vi "movement forward by santimeters.vi"() -> ()   [LabVIEW 2017]
uses:
  <vilib>/myRIO/Common/Instrument Driver Framework/Utilities/typedefs/FPGA Ref Manager Action Enum.ctl
  <vilib>/myRIO/Common/Instrument Driver Framework/myRIO v1.0/Encoder/typedefs/Encoder Signal Mode.ctl
  <vilib>/myRIO/Instrument Drivers/Onboard IO/Encoder/typedefs/Encoder Reference.ctl
  <vilib>/myRIO/Common/Instrument Driver Framework/Utilities/typedefs/myRIO Generic Hardware Reference.ctl
  <vilib>/myRIO/Common/Instrument Driver Framework/Utilities/typedefs/Hardware Version Enum.ctl
  <vilib>/myRIO/Common/Instrument Driver Framework/Utilities/typedefs/myRIO v1.0 Reference.ctl
  <vilib>/myRIO/Common/Instrument Driver Framework/Utilities/typedefs/Generic FPGA Reference.ctl
  <vilib>/myRIO/Common/Instrument Driver Framework/myRIO v1.0/Encoder/typedefs/Encoder Channels Enum.ctl
  <vilib>/myRIO/Common/Instrument Driver Framework/myRIO v1.0/Encoder/typedefs/Encoder Configuration v1.0.ctl
  <vilib>/userdefined/High Color/nirio_resource_hc.ctl
  <vilib>/myRIO/Instrument Drivers/Onboard IO/I2C/typedefs/I2C Reference.ctl
  <vilib>/myRIO/Common/Instrument Driver Framework/myRIO v1.0/I2C/typedefs/I2C Channels Enum.ctl
  <vilib>/myRIO/Instrument Drivers/Onboard IO/I2C/typedefs/I2C Configuration.ctl
  <vilib>/myRIO/Instrument Drivers/Onboard IO/I2C/typedefs/I2C Transfer Rate.ctl
  <vilib>/myRIO/Common/Instrument Driver Framework/Utilities/vis/Is FPGA Ref Available.vi
  <vilib>/myRIO/Common/Instrument Driver Framework/myRIO v1.0/Encoder/vis/myRIO v1.1 Open Encoder.vi
  <vilib>/myRIO/Instrument Drivers/Onboard IO/Encoder/vis/Read.vi
  <vilib>/myRIO/Common/Instrument Driver Framework/myRIO v1.0/I2C/vis/myRIO v1.1 Open I2C.vi
  <vilib>/myRIO/Common/Instrument Driver Framework/Utilities/vis/Validate Channels.vi
  <vilib>/myRIO/Common/Instrument Driver Framework/myRIO v1.0/Encoder/vis/myRIO v1.0 Reserve Encoder.vi
  <vilib>/myRIO/Common/Instrument Driver Framework/myRIO v1.0/I2C/vis/myRIO v1.0 Reserve I2C.vi
  <vilib>/myRIO/Common/Instrument Driver Framework/myRIO v1.0/I2C/vis/myRIO v1.0 Close I2C.vi
  <vilib>/myRIO/Common/Instrument Driver Framework/myRIO v1.0/Encoder/vis/myRIO v1.0 Build MUX Configuration Encoder.vi
  <vilib>/myRIO/Common/Instrument Driver Framework/myRIO v1.0/Resource Manager/vis/myRIO v1.0 Reserve Channel List.vi
  <vilib>/myRIO/Common/Instrument Driver Framework/myRIO v1.0/I2C/vis/myRIO v1.0 Build MUX Configuration I2C.vi
  <vilib>/myRIO/Common/Instrument Driver Framework/myRIO v1.0/I2C/vis/myRIO v1.0 Unreserve I2C.vi
  <vilib>/myRIO/Common/Instrument Driver Framework/myRIO v1.0/Resource Manager/vis/myRIO v1.0 Create Configuration List.vi
  <vilib>/myRIO/Common/Instrument Driver Framework/myRIO v1.0/Resource Manager/vis/myRIO v1.0 Reserve Channel.vi
  <vilib>/myRIO/Common/Instrument Driver Framework/myRIO v1.0/Resource Manager/vis/myRIO v1.0 Unreserve Channel.vi
  <vilib>/myRIO/Common/Instrument Driver Framework/myRIO v1.0/Resource Manager/vis/myRIO v1.0 Unreserve Channel List.vi
  <vilib>/myRIO/Common/Instrument Driver Framework/myRIO v1.0/Resource Manager/vis/myRIO v1.0 Build Mutex Name.vi
  <vilib>/Utility/VariantDataType/GetNumericInfo.vi
  <vilib>/Utility/error.llb/Error Cluster From Error Code.vi
  <vilib>/myRIO/Common/Instrument Driver Framework/myRIO v1.0/myRIO v1.1 Open.vi
  <vilib>/myRIO/Common/Instrument Driver Framework/Utilities/vis/IO Manager.vi
  <vilib>/myRIO/Common/Instrument Driver Framework/Utilities/vis/Configuration Manager.vi
  <vilib>/myRIO/Common/Instrument Driver Framework/myRIO v1.0/Resource Manager/vis/myRIO v1.0 Configure IO.vi
  <vilib>/myRIO/Common/Instrument Driver Framework/myRIO v1.0/myRIO v1.0 Close.vi
  <vilib>/myRIO/Common/Instrument Driver Framework/myRIO v1.0/Encoder/vis/myRIO v1.0 Configure Encoder.vi
  <vilib>/myRIO/Common/Instrument Driver Framework/myRIO v1.0/Encoder/vis/myRIO v1.0 Read Encoder.vi
  <vilib>/myRIO/Common/Instrument Driver Framework/myRIO v1.0/I2C/vis/myRIO v1.0 Shutdown I2C.vi
  <vilib>/myRIO/Instrument Drivers/Onboard IO/I2C/vis/myRIO I2C Open.xnode
  <vilib>/myRIO/Express VI/Onboard IO/Encoder/Encoder Express VI.xnode
  <vilib>/myRIO/Instrument Drivers/Onboard IO/Encoder/vis/myRIO Encoder Open.xnode
  <vilib>/myRIO/Instrument Drivers/Onboard IO/I2C/I2C.lvlib
  <vilib>/myRIO/Instrument Drivers/Onboard IO/Encoder/Encoder.lvlib
panel:
  in  "range in santimeters":dbl format="%#_13g"
  out "main angle":ext
  out "error out":errorcluster
  in  "error in (no error)":errorcluster
  out "axis Z(after)":ext
  out "zero angle":ext
  out "left":dbl
  out "right":dbl
  out "axis Z(paste)":ext
  in  "Stop Button":bool
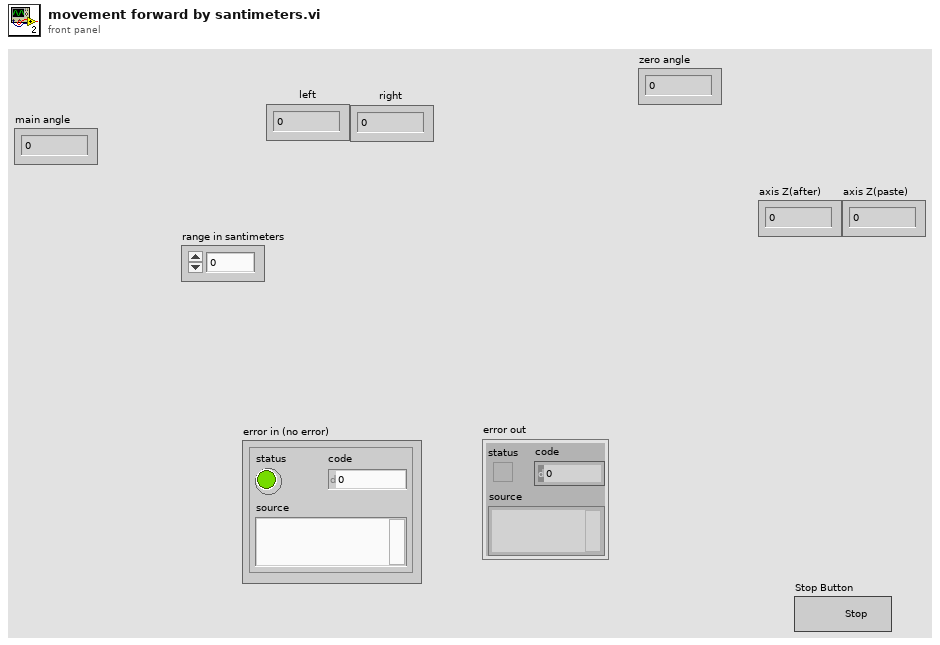
[diagram p1: front panel]
types:
  T1 = typedef "FPGA Ref Manager Action Enum.ctl" = enum16{"Get", "Set", "Reset"}
  T2 = typedef "I2C.lvlib/I2C Reference.ctl" = cluster{"myRIO Reference":T3, "I2C Channels Enum":T7, "I2C Configuration":T8}
  T3 = typedef "myRIO Generic Hardware Reference.ctl" = cluster{"myRIO Model":T4, "myRIO Hardware Reference":T5}
  T4 = typedef "Hardware Version Enum.ctl" = enum16{"Unknown", "myRIO-1900", "myRIO-1950", "roboRIO", "NI ELVIS RIO CM"}
  T5 = typedef "myRIO v1.0 Reference.ctl" = cluster{"Generic FPGA Reference":T6, "Allow multiple opens":bool}
  T6 = typedef "Generic FPGA Reference.ctl" = refnum<k20>
  T7 = typedef "I2C Channels Enum.ctl" = enum16{"Not Connected", "A/I2C", "B/I2C", "I2C/I2C"}
  T8 = typedef "I2C.lvlib/I2C Configuration.ctl" = cluster{"I2C Transfer Rate":T9}
  T9 = typedef "I2C.lvlib/I2C Transfer Rate.ctl" = enum16{"Standard mode (100 kbps)", "Fast mode (400 kbps)"}
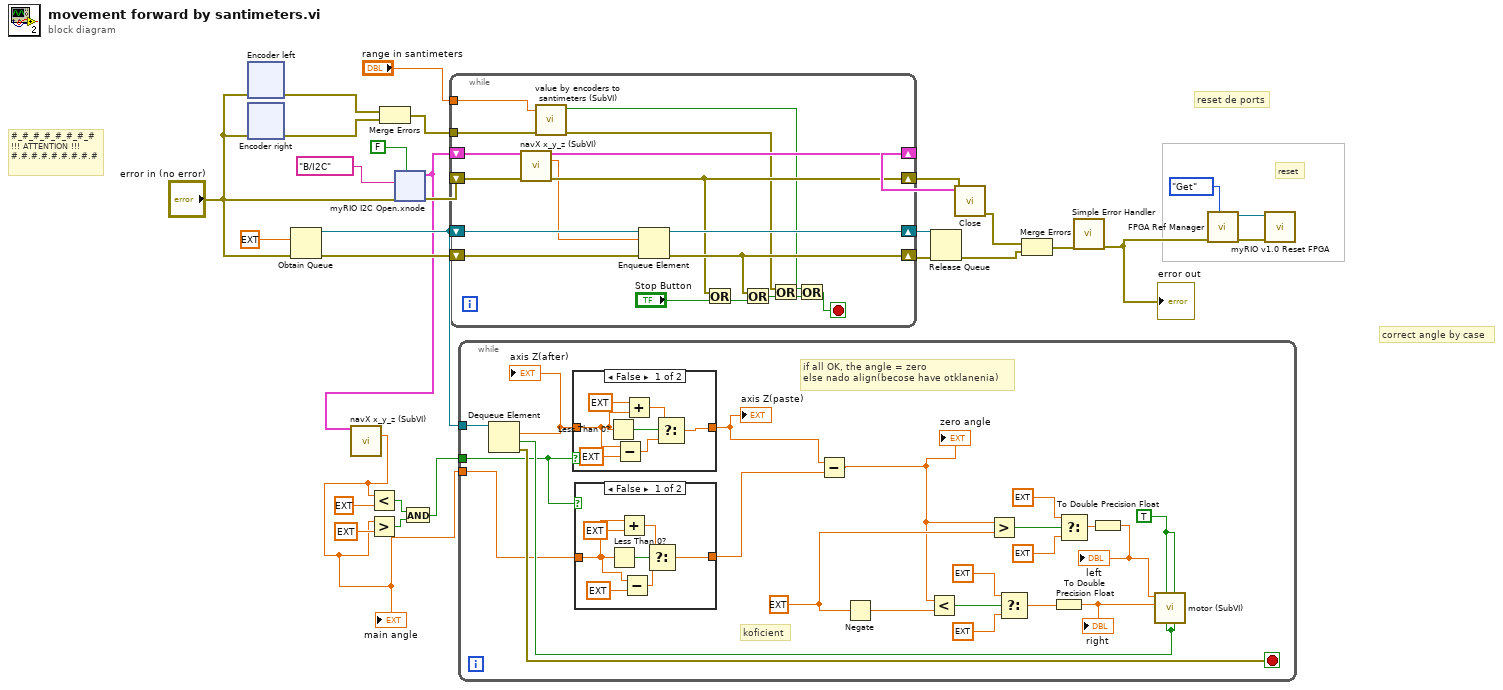
[diagram p0: block diagram]
diagram:
  # "correct angle by case"
  # "reset de ports"
  # "#_#_#_#_#_#_#_#\n!!! ATTENTION !!!\n#.#.#.#.#.#.#.#.#"
  # "reset"
  n1 = xnode ("Encoder left")("error in (no error)"="error in (no error)") -> ("error out"=w4:errorcluster)  [unwired: 1 in, 3 out]
  n2 = xnode ("Encoder right")("error in (no error)"="error in (no error)") -> ("error out"=w3:errorcluster)  [unwired: 1 in, 3 out]
  n3 = Obtain Queue(element data type=ext 0.0 ("value Z"), error in (no error)="error in (no error)") -> (queue out=w17:refnum<queue>, error out=w29:errorcluster)  [unwired: 3 in, 1 out]
  n4 = Merge Errors(w4, w3) -> (w2:errorcluster)
  n5 = xnode "myRIO I2C Open.xnode"("error in (no error)"="error in (no error)", "Allow multiple opens?"=FALSE, "Channel Name"=tag "B/I2C") -> ("error out"=w22:errorcluster, "I2C Ref Out"=w13:T2)
  n6 = call "navX x_y_z (SubVI).vi"("I2C Ref Out in"=w13) -> ("value Z"=w10:ext)  [unwired: 10 in, 4 out]
  "main angle" <- w10
  n7 = Less?(x=w10, y=ext 90.0) -> (x < y?=w8:bool)
  n8 = Greater?(x=w10, y=ext -90.0) -> (0:w11:bool)
  n9 = And(x=w8, y=w11) -> (x .and. y?=w7:bool)
  n10 = while {
    shift-right: [w41] -> w27
    shift-left: w29 -> [w46]
    shift-right: [w45] -> w28
    shift-left: w17 -> [w47]
    shift-right: [w42] -> w23
    shift-left: w13 -> [w43]
    shift-right: [w38] -> w21
    shift-left: w22 -> [w39]
    tunnel: w2 -> [w33]
    tunnel: "range in santimeters" -> [w31]
    stop <- w35 stop-if-true
    n11 = call "navX x_y_z (SubVI).vi"("I2C Ref Out in"=w43, "error in (no error)"=w39) -> ("I2C Ref Out out"=w42:T2, "value Z"=w37:ext, "error out"=w38:errorcluster)  [unwired: 9 in, 2 out]
    n12 = call "value by encoders to santimeters (SubVI).vi"("error in (no error)"=w33, "range in"=w31) -> ("error out"=w32:errorcluster, "value >= range"=w30:bool)  [unwired: 7 in, 1 out]
    n13 = Enqueue Element(queue=w47, element=w37, error in (no error)=w46) -> (queue out=w45:refnum<queue>, error out=w41:errorcluster)  [unwired: 1 in, 1 out]
    n14 = Or(x=w38, y="Stop Button") -> (x .or. y?=w40:bool)
    n15 = Or(x=w41, y=w40) -> (x .or. y?=w36:bool)
    n16 = Or(x=w32, y=w36) -> (x .or. y?=w34:bool)
    n17 = Or(x=w30, y=w34) -> (x .or. y?=w35:bool)
  }
  n18 = while {
    tunnel: w17 -> [w69]
    tunnel: w10 -> [w51]
    tunnel: w7 -> [w50]
    stop <- w68 stop-if-true
    w57 = TRUE ("M0 (Pin 21)")
    w61 = ext 1.0 ("y")
    # "koficient"
    # "if all OK, the angle = zero\nelse nado align(becose have otklanenia)"
    n19 = Dequeue Element(queue=w69) -> (element=w53:ext, timed out?=w56:bool, error out=w68:errorcluster)  [unwired: 2 in, 1 out]
    "axis Z(after)" <- w53
    n20 = case shown="False" w50 {
      tunnel: [w83 w85] -> w54
      tunnel: w53 -> [w79 w85]
      frame False {
        n21 = Less Than 0?(x=w79) -> (x < 0?=w84:bool)
        n22 = Subtract(x=w79, y=ext 180.0) -> (x-y=w80:ext)
        n23 = Add(x=ext 180.0, y=w79) -> (x+y=w82:ext)
        n24 = Select(t=w82, s=w84, f=w80) -> (s? t:f=w83:ext)
      }
      frame True {
      }
    }
    "axis Z(paste)" <- w54
    n25 = case shown="False" w50 {
      tunnel: [w75 w77] -> w52
      tunnel: w51 -> [w72 w77]
      frame False {
        n26 = Less Than 0?(x=w72) -> (x < 0?=w76:bool)
        n27 = Add(x=w72, y=ext 180.0) -> (x+y=w74:ext)
        n28 = Subtract(x=w72, y=ext 180.0) -> (x-y=w73:ext)
        n29 = Select(t=w74, s=w76, f=w73) -> (s? t:f=w75:ext)
      }
      frame True {
      }
    }
    n30 = Subtract(x=w54, y=w52) -> (x-y=w55:ext)
    "zero angle" <- w55
    n31 = Negate(x=w61) -> (-x=w60:ext)
    n32 = Less?(x=w55, y=w60) -> (x < y?=w64:bool)
    n33 = Greater?(x=w55, y=w61) -> (0:w67:bool)
    n34 = Select(t=ext 0.2 ("y"), s=w64, f=ext 0.4 ("y")) -> (s? t:f=w58:ext)
    n35 = To Double Precision Float(number=w58) -> (double precision float=w49:dbl)
    "right" <- w49
    n36 = Select(t=ext 0.2 ("y"), s=w67, f=ext 0.4 ("y")) -> (s? t:f=w59:ext)
    n37 = To Double Precision Float(number=w59) -> (double precision float=w48:dbl)
    "left" <- w48
    n38 = call "motor (SubVI).vi"("M1 (Pin 26)"=w56, "M1 (Pin 25)"=w57, "M0 (Pin 23)"=w56, "M0 (Pin 21)"=w57, "PWM1"=w49, "PWM0"=w48) -> ()  [unwired: 5 in, 1 out]
  }
  n39 = Release Queue(queue=w28, error in (no error)=w27) -> (error out=w18:errorcluster)  [unwired: 1 in, 2 out]
  n40 = call <vilib>:"Close.vi"("error in (no error)"=w21, "I2C Ref In"=w23) -> ("error out"=w19:errorcluster)  [unwired: 9 in]
  n41 = Merge Errors(w19, w18) -> (w20:errorcluster)
  n42 = call <vilib>:"Simple Error Handler.vi"("error in (no error)"=w20) -> ("error out"=w14:errorcluster)  [unwired: 4 in, 4 out]
  "error out" <- w14
  n43 = call <vilib>:"FPGA Ref Manager.vi"("Action"=FPGA_Ref_Manager_Action_Enum."Get" ("Ref Counter Action Enum"), "error in (no error)"=w14) -> ("error out"=w6:errorcluster, "Generic FPGA Reference out"=w16:T6)  [unwired: 7 in]
  n44 = call <vilib>:"myRIO v1.0 Reset FPGA.vi"("error in (no error)"=w6, "Generic FPGA Reference in"=w16) -> ()  [unwired: 8 in, 2 out]
